vi "testWaveform.vi"(8 "error in (no error)":errorcluster, 11 "TestCase in":refnum<class "EasyXMLTest.lvclass">) -> (0 "error out":errorcluster, 3 "TestCase out":refnum<class "EasyXMLTest.lvclass">)   [LabVIEW 2011, in "EasyXMLTest.lvclass"]
doc: "Verify that error in is not overwritten"
uses:
  EasyXMLTest.lvclass
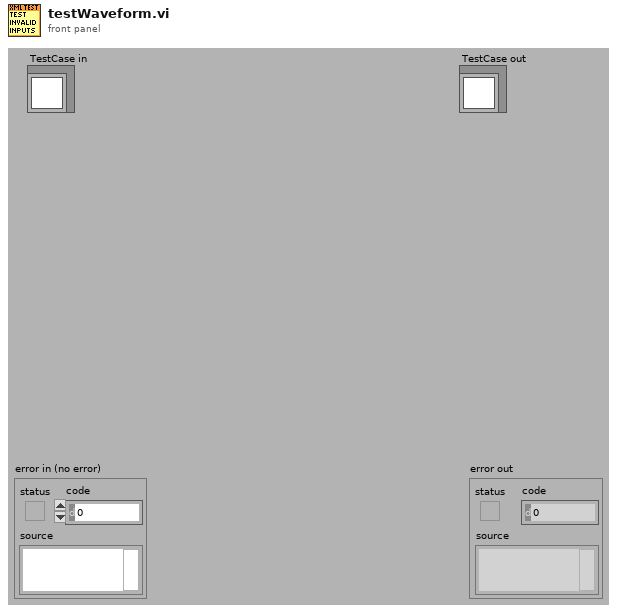
[diagram p1: front panel]
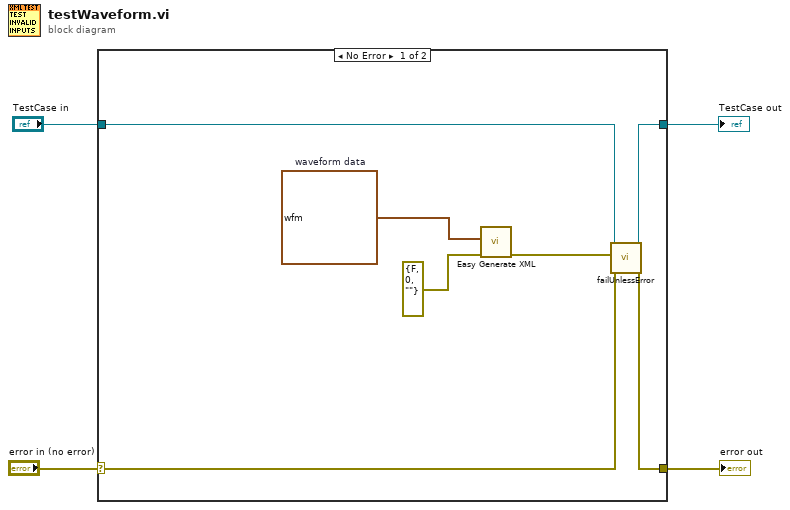
[diagram p0: block diagram]
diagram:
  n1 = case shown="No Error" "error in (no error)" {
    selector: "error in (no error)" -> [w7 w13]
    tunnel: [w6 w13] -> w2
    tunnel: [w11 w12] -> w1
    tunnel: "TestCase in" -> [w8 w12]
    frame No Error {
      w10 = waveform(dbl) {"t0"=timestamp(0 s since 1904-01-01), "dt"=1.0, "Y"=[]}  # waveform data
      n2 = call "Easy Generate XML.vi"("error in (no error)"=errorcluster {"status"=FALSE, "code"=0, "source"=""}, "LabVIEW Data"=w10) -> ("error out"=w9:errorcluster)  [unwired: 8 in, 1 out]
      n3 = call-dynamic "failUnlessError.vi"("error in (no error)"=w7, "error"=w9, "TestCase in"=w8) -> ("error out"=w6:errorcluster, "TestCase out"=w11:refnum<class "EasyXMLTest.lvclass">)  [unwired: 7 in]
    }
    frame Error {
    }
  }
  "error out" <- w2
  "TestCase out" <- w1
